vi "zest_5_part_1.vi"() -> ()   [LabVIEW 2023]
panel:
  out "element 8":bool
  out "element 7":bool
  out "element 6":bool
  out "element 5":bool
  out "element 4":bool
  out "element 3":bool
  out "element 2":bool
  out "element":bool
  in  "Enum":enum16{"", "AND", "OR", "XOR"}(ring)
  in  "stop":bool
  in  "?":bool
  in  "?":bool
  in  "?":bool
  in  "?":bool
  in  "?":bool
  in  "?":bool
  in  "?":bool
  in  "?":bool
  in  "?":bool
  in  "?":bool
  in  "?":bool
  in  "?":bool
  in  "?":bool
  in  "?":bool
  in  "?":bool
  in  "?":bool
  in  "?":bool
  in  "?":bool
  in  "?":bool
  in  "?":bool
  in  "?":bool
  in  "?":bool
  in  "?":bool
  in  "?":bool
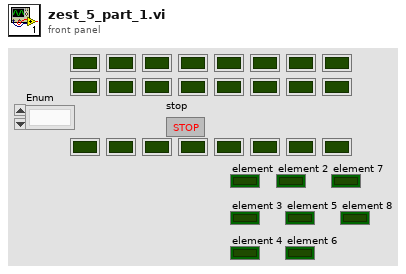
[diagram p1: front panel]
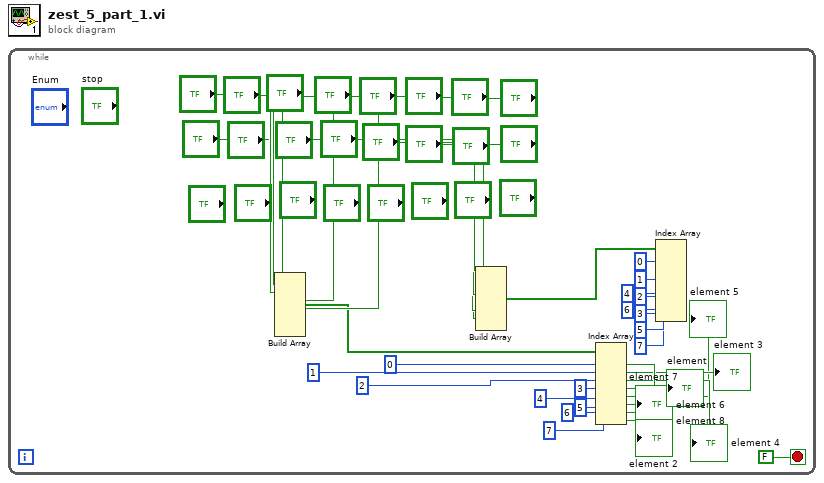
[diagram p0: block diagram]
diagram:
  n1 = while {
    stop <- FALSE stop-if-true
    n2 = Build Array("?", "?", "?", "?", "?", "?", "?", "?") -> (w28:bool[])
    n3 = Build Array("?", "?", "?", "?", "?", "?", "?", "?") -> (w18:bool[])
    n4 = Index Array(array=w28, index #1=0 ("index"), index #2=1 ("index"), index #3=2 ("index"), index #4=3 ("index"), index #5=4 ("index"), index #6=5 ("index"), index #7=6 ("index"), index #8=7 ("index")) -> (element #1=→"element 2":bool, element #2=→"element 3":bool, element #3=→"element 4":bool, element #4=→"element":bool, element #5=→"element 5":bool, element #6=→"element 6":bool, element #7=→"element 7":bool, element #8=→"element 8":bool)
    n5 = Index Array(array=w18, index #1=0 ("index"), index #2=1 ("index"), index #3=2 ("index"), index #4=3 ("index"), index #5=4 ("index"), index #6=5 ("index"), index #7=6 ("index"), index #8=7 ("index")) -> ()  [unwired: 8 out]
  }
